vi "Write A-V and Publish.vi"(6 "measurement":dbl format="%^.2e", 8 "error in (no error)":errorcluster, 9 "measurement type (voltage)":i32(ring)=1 items=["Voltage"=1, "Current"=0], 10 "channel name (\"CHANNEL1\")":string="CHANNEL1", 11 "CS++DCPwr in":refnum<class "CS++DCPwr.lvclass">) -> (0 "error out":errorcluster, 3 "CS++DCPwr out":refnum<class "CS++DCPwr.lvclass">)   [LabVIEW 2013, in "CS++DCPwr.lvlib" / "CS++DCPwr.lvclass"]
doc: "Write measurement value to attribute and publish to PV."
uses:
  CS++DCPwr.lvclass
  Core/Classes/CS++ProcessVariables/ProcessVariable/PV.lvclass
  CS++DCPwr.lvclass/CS++DCPwr.ctl
  Core/Classes/CS++ProcessVariables/PVConnection/PVConnection.lvclass
  Core/Classes/CS++ProcessVariables/ProcessVariable/PV.lvclass/PV.ctl
  Core/Classes/CS++ProcessVariables/ProcessVariable/Write Data.vi
  Core/Classes/CS++ProcessVariables/ProcessVariable/Write Timestamp.vi
  Core/Classes/CS++ProcessVariables/ProcessVariable/Write Error.vi
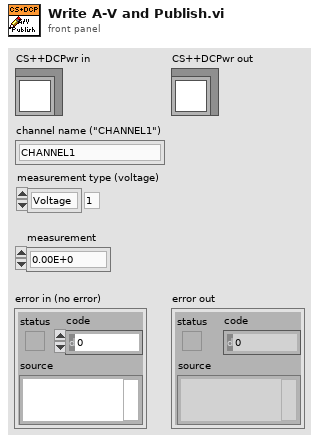
[diagram p1: front panel]
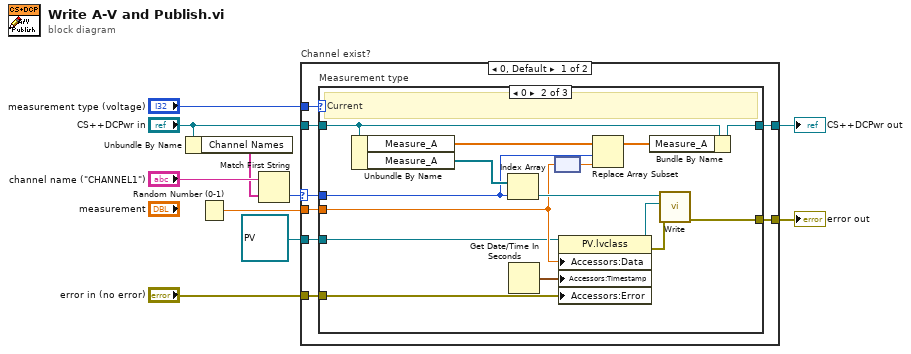
[diagram p0: block diagram]
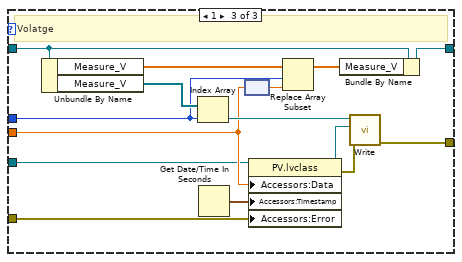
[diagram p3: hidden frame]
diagram:
  n1 = Unbundle By Name("CS++DCPwr in") -> ("Channel Names"=w6:string[])
  n2 = Random Number (0-1)() -> (number: 0 to 1=w1:dbl)
  n3 = Match First String(2:w6, 3:"channel name (\"CHANNEL1\")") -> (0:w5:i32)  [unwired: 1 out]
  n4 = case "Channel exist?" shown="0, Default" w5 {
    selector: w5 -> [w14 _]
    tunnel: [w17 w52] -> w9
    tunnel: "CS++DCPwr in" -> [w16 w52]
    tunnel: "measurement type (voltage)" -> [w18 _]
    tunnel: w1 -> [w15 _]
    tunnel: "error in (no error)" -> [w13 w51]
    tunnel: [w12 w51] -> w3
    tunnel: refnum<class "PV.lvclass"> refnum ("PV") -> [w11 _]
    frame 0, Default {
      n5 = case "Measurement type" shown="0" w18 {
        tunnel: [w20 w34 w49] -> w17
        tunnel: w16 -> [w20 w35 w50]
        tunnel: w15 -> [_ w27 w42]
        tunnel: w14 -> [_ w24 w39]
        tunnel: w13 -> [w19 w23 w38]
        tunnel: [w19 w22 w37] -> w12
        tunnel: w11 -> [_ w21 w36]
        frame Default {
        }
        frame 0 {
          # "Current"
          n6 = Unbundle By Name(w35) -> ("Measure_A"=w33:dbl[unit][], "Measure_A"=w30:refnum<class "PVConnection.lvclass">[])
          n7 = Index Array(array=w30, index=w24) -> (element=w29:refnum<class "PVConnection.lvclass">)
          n8 = Get Date/Time In Seconds() -> (seconds since 1Jan1904=w25:timestamp)
          n9 = node(w27) -> (w31:dbl[unit])
          n10 = property class="PV.lvclass"(reference=w21, "Accessors:Data"=w27, "Accessors:Timestamp"=w25, "Accessors:Error"=w23) -> (reference out=w28:refnum<class "PV.lvclass">, error out=w26:errorcluster)  [unwired: 1 in]
          n11 = Replace Array Subset(array=w33, new element=w31, index=w24) -> (w32:dbl[unit][])
          n12 = Bundle By Name(cluster=w35, "Measure_A"=w32) -> (w34:refnum<class "CS++DCPwr.lvclass">)
          n13 = call-dynamic "Write.vi"("error in (no error)"=w26, "PV"=w28, "PVConnection in"=w29) -> ("error out"=w22:errorcluster)  [unwired: 7 in, 1 out]
        }
        frame 1 {
          # "Volatge"
          n14 = Unbundle By Name(w50) -> ("Measure_V"=w48:dbl[unit][], "Measure_V"=w45:refnum<class "PVConnection.lvclass">[])
          n15 = Index Array(array=w45, index=w39) -> (element=w44:refnum<class "PVConnection.lvclass">)
          n16 = Get Date/Time In Seconds() -> (seconds since 1Jan1904=w40:timestamp)
          n17 = node(w42) -> (w46:dbl[unit])
          n18 = property class="PV.lvclass"(reference=w36, "Accessors:Data"=w42, "Accessors:Timestamp"=w40, "Accessors:Error"=w38) -> (reference out=w43:refnum<class "PV.lvclass">, error out=w41:errorcluster)  [unwired: 1 in]
          n19 = Replace Array Subset(array=w48, new element=w46, index=w39) -> (w47:dbl[unit][])
          n20 = Bundle By Name(cluster=w50, "Measure_V"=w47) -> (w49:refnum<class "CS++DCPwr.lvclass">)
          n21 = call-dynamic "Write.vi"("error in (no error)"=w41, "PV"=w43, "PVConnection in"=w44) -> ("error out"=w37:errorcluster)  [unwired: 7 in, 1 out]
        }
      }
    }
    frame -1 {
    }
  }
  "error out" <- w3
  "CS++DCPwr out" <- w9
